vi "SW_Type_1a_correction.vi"(1 "Tmeas (degC)":dbl, 2 "Calib consts.":dbl[](array[numeric])) -> (0 "Corrected calib consts.":dbl[](array[numeric]))   [LabVIEW 2011]
panel:
  # "Type 1a: Open ended. Single calibration corrected to conditions at t"
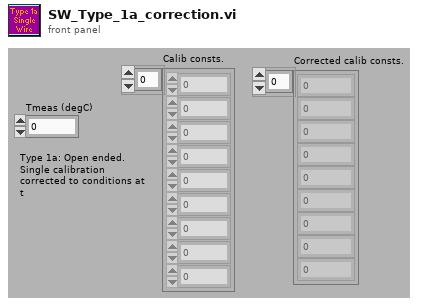
[diagram p1: front panel]
types:
  T1 = cluster{"Calib consts.[0]":dbl, "Calib consts.[1]":dbl, "Calib consts.[2]":dbl, "Calib consts.[3]":dbl, "Calib consts.[4]":dbl, "Calib consts.[5]":dbl, "Calib consts.[6]":dbl, "Calib consts.[7]":dbl}
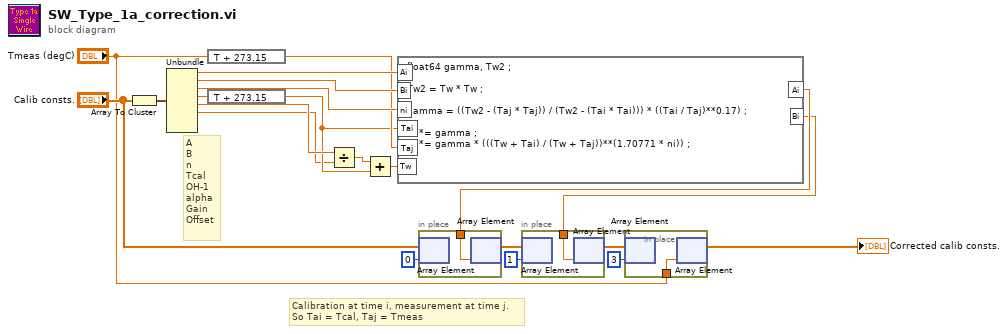
[diagram p0: block diagram]
diagram:
  # "Calibration at time i, measurement at time j.\nSo Tai = Tcal, Taj = Tmeas"
  # "A\nB\nn\nTcal\nOH-1\nalpha\nGain\nOffset"
  n1 = Array To Cluster(array="Calib consts.") -> (cluster=w21:T1)
  n2 = Unbundle(w21) -> ("Calib consts.[0]"=w20:dbl, "Calib consts.[1]"=w19:dbl, "Calib consts.[2]"=w18:dbl, "Calib consts.[3]"=w13:dbl, "Calib consts.[4]"=w17:dbl, "Calib consts.[5]"=w1:dbl)  [unwired: 2 out]
  n3 = expression code="T + 273.15"("Tmeas (degC)") -> (w14:dbl)
  n4 = expression code="T + 273.15"(w13) -> (w12:dbl)
  n5 = Divide(x=w17, y=w1) -> (x/y=w10:dbl)
  n6 = Add(x=w10, y=w12) -> (x+y=w9:dbl)
  n7 = formula code="float64 gamma, Tw2 ;\n\nTw2 = Tw * Tw ;\n\ngamma = ((Tw2 - (Taj * Taj)) / (Tw2 - (Tai * Tai))) * ((Tai / Taj)**0.17) ;\n\nAi *= gamma ;\nBi *= gamma * (((Tw + Tai) / (Tw + Taj))**(1.70771 * ni)) ;"("Ai"=w20, "Bi"=w19, "ni"=w18, "Tai"=w12, "Taj"=w14, "Tw"=w9) -> ("Ai"=w7:dbl, "Bi"=w6:dbl)
  n8 = in-place {
    in-place-border: w7 -> [w22]
    n9 = in-place-array #1("Calib consts.", 0) -> ()  [unwired: 1 out]
    n10 = in-place-array #1(w22) -> (w4:dbl[])  [unwired: 1 out]
  }
  n11 = in-place {
    in-place-border: w6 -> [w23]
    n12 = in-place-array #2(w4, 1) -> ()  [unwired: 1 out]
    n13 = in-place-array #2(w23) -> (w2:dbl[])  [unwired: 1 out]
  }
  n14 = in-place {
    in-place-border: "Tmeas (degC)" -> [w24]
    n15 = in-place-array #3(w2, 3) -> ()  [unwired: 1 out]
    n16 = in-place-array #3(w24) -> (→"Corrected calib consts.":dbl[])  [unwired: 1 out]
  }
